vi "MyGraph-Facade.vi"(0 "Data In":T4, 2 "Display State In":T2, 3 "Container State":T3) -> (6 "Data Out":T4, 7 "Display State Out":T2, 8 "Action":T1)   [LabVIEW 2015, in "MyGraph.xctl"]
uses:
  MyGraph.xctl
  MyGraph-Data.ctl
  <vilib>/_xctls/Container State.ctl
  MyGraph-State.ctl
  <vilib>/_xctls/Action.ctl
  <vilib>/_xctls/XControlSupport.lvlib
panel:
  in  "ZoomREC":bool
  in  "ZoomToFit":bool
  in  "ZoomOut":bool
  in  "ZoomIn":bool
  in  "ZoomY":bool
  in  "ZoomX":bool
  in  "Select":bool
  out "Waveform Graph":waveform(dbl)[](graph)
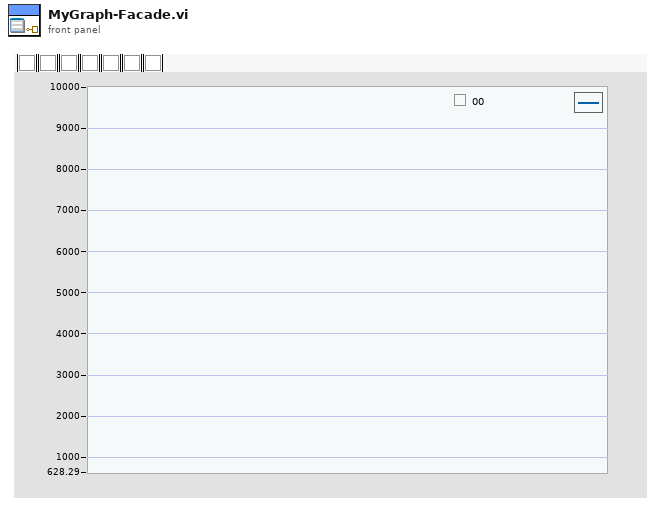
[diagram p1: front panel]
types:
  T1 = typedef "XControlSupport.lvlib/Action.ctl" = cluster{"Data Changed?":bool, "State Changed?":bool, "Action Name":string}
  T2 = typedef "MyGraph.xctl/MyGraph-State.ctl" = cluster{"PlotNames":string[], "event registration refnum":refnum<event-registration>}
  T3 = typedef "XControlSupport.lvlib/Container State.ctl" = cluster{"Indicator?":bool, "Run Mode?":bool, " Refnum":refnum<vi>}
  T4 = typedef "MyGraph.xctl/MyGraph-Data.ctl" = waveform(dbl)[]
  T5 = cluster{"ActTool":i32, "EmptyImg":picture, "StartPoints":cluster{i16, i16}[]}
  T6 = typedef "LVPoint32TypeDef.ctl" = cluster{"Horizontal":i32, "Vertical":i32}
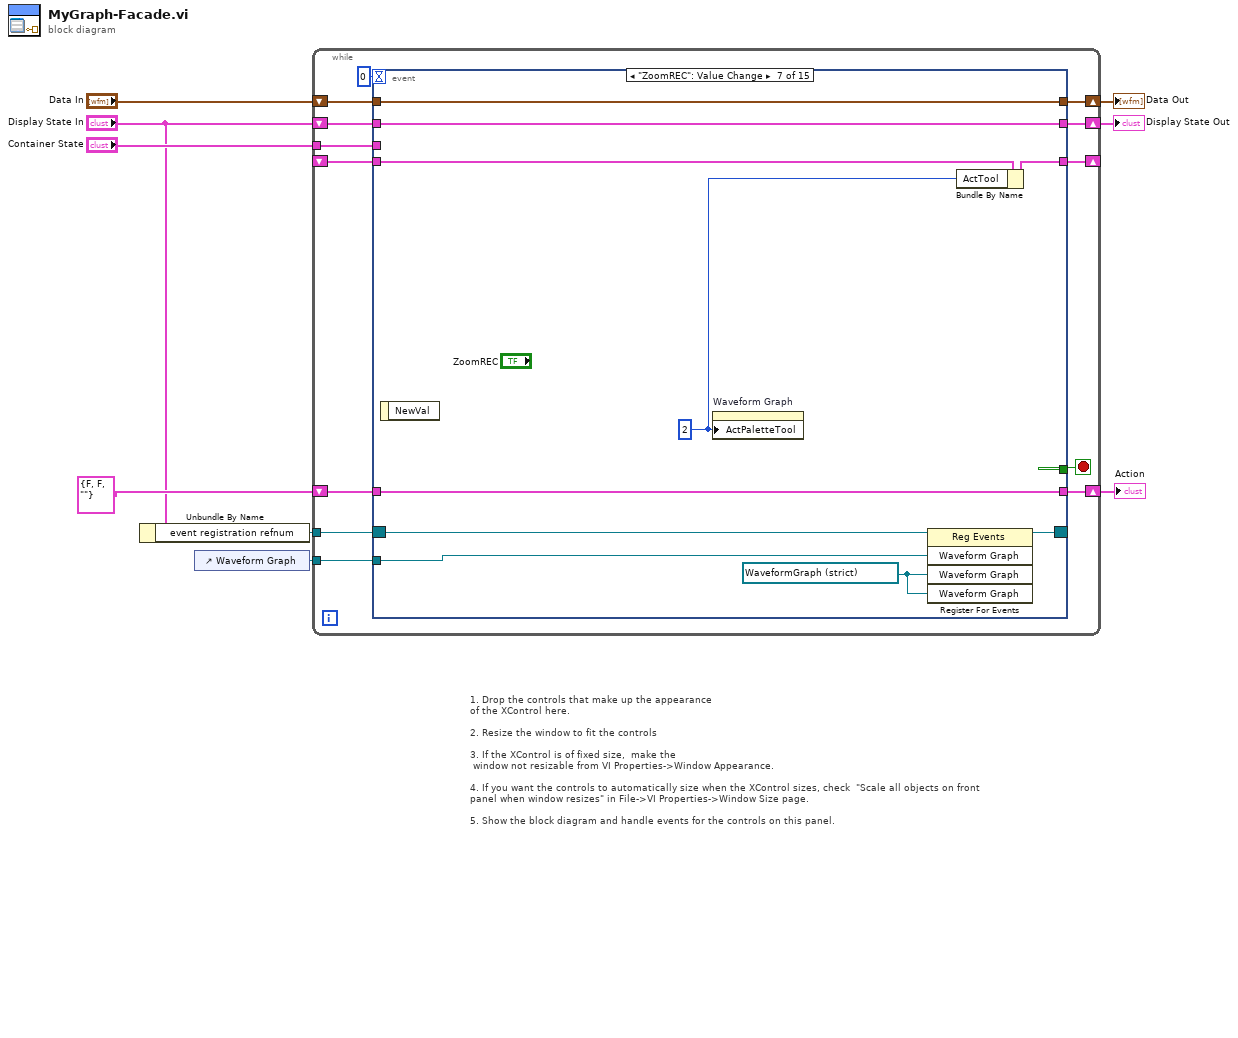
[diagram p0: block diagram]
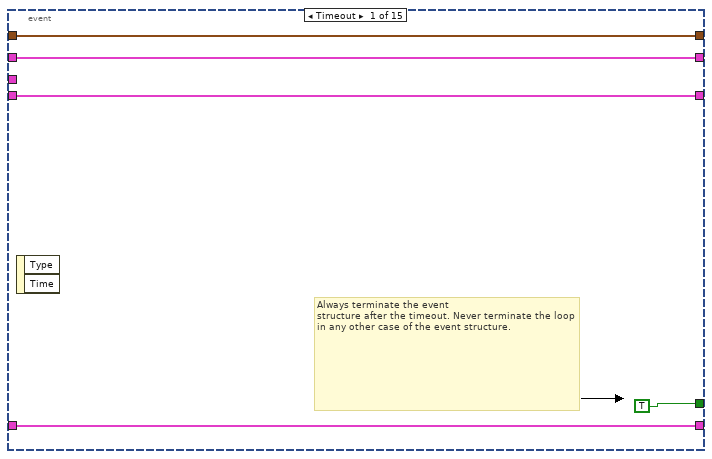
[diagram p2: hidden frame]
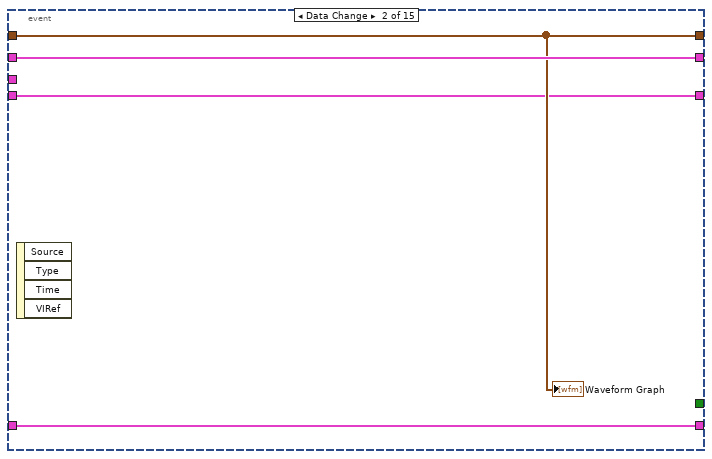
[diagram p3: hidden frame]
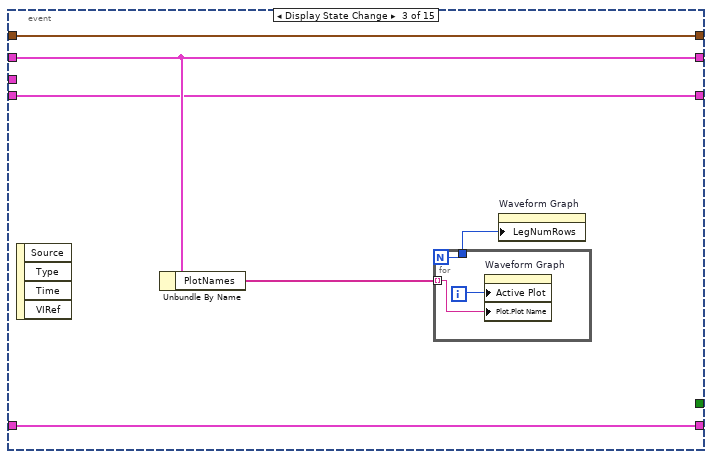
[diagram p4: hidden frame]
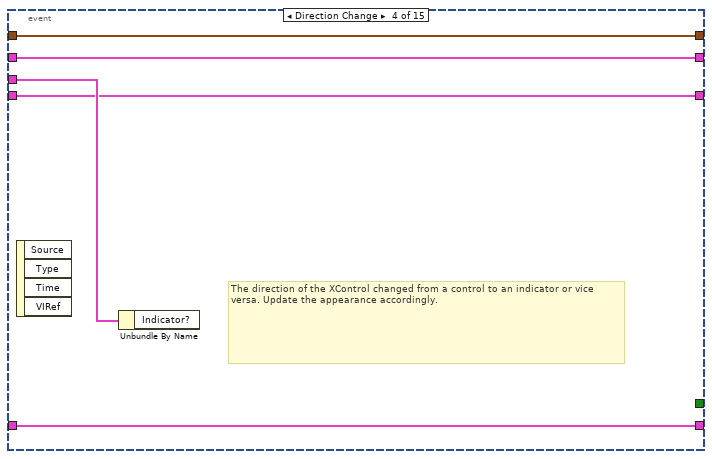
[diagram p5: hidden frame]
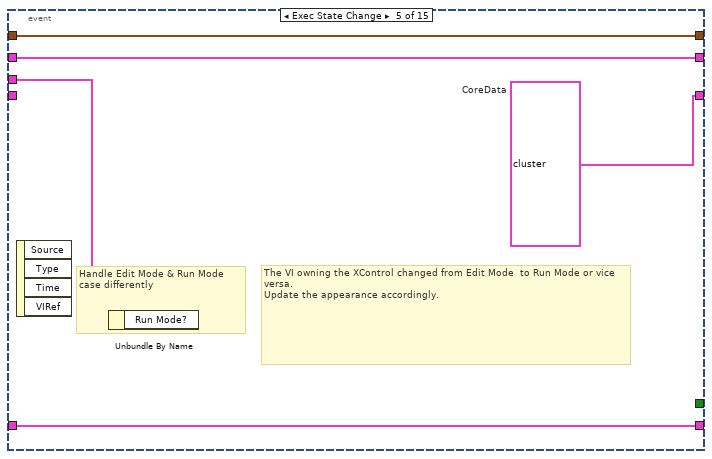
[diagram p6: hidden frame]
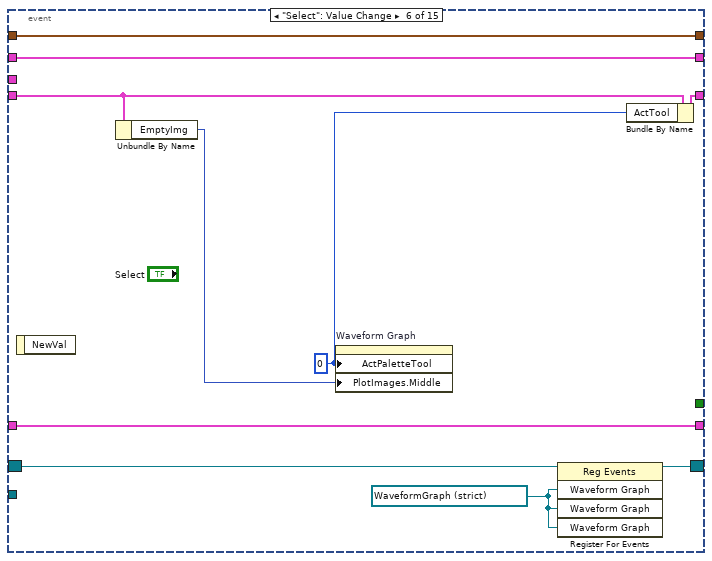
[diagram p7: hidden frame]
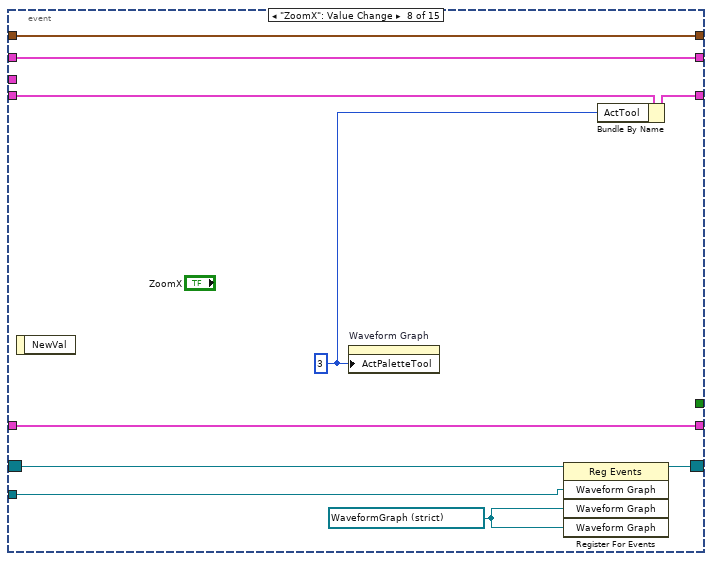
[diagram p8: hidden frame]
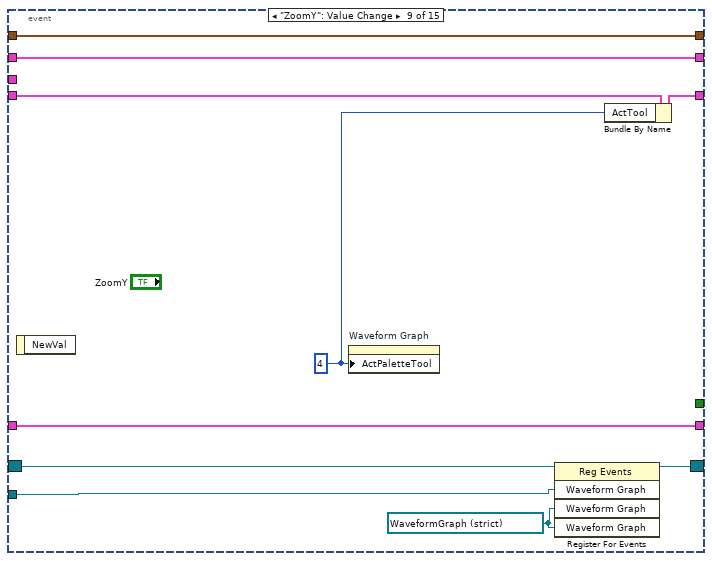
[diagram p9: hidden frame]
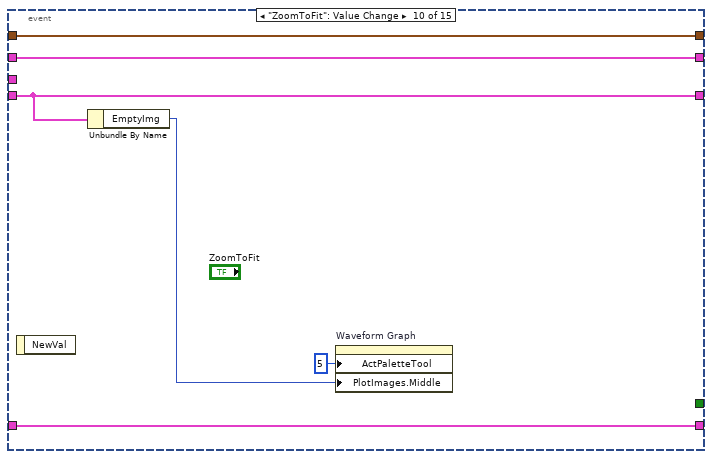
[diagram p10: hidden frame]
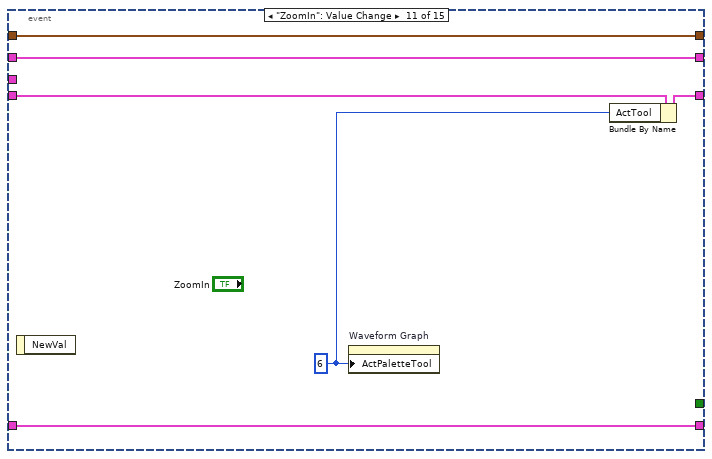
[diagram p11: hidden frame]
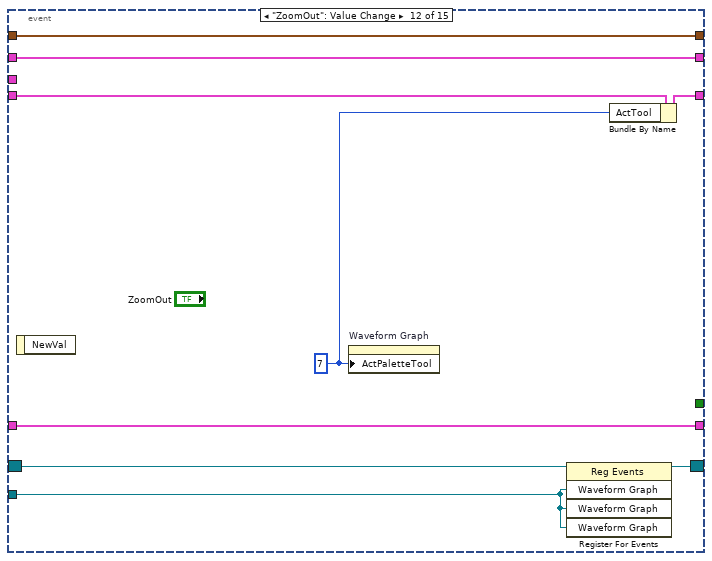
[diagram p12: hidden frame]
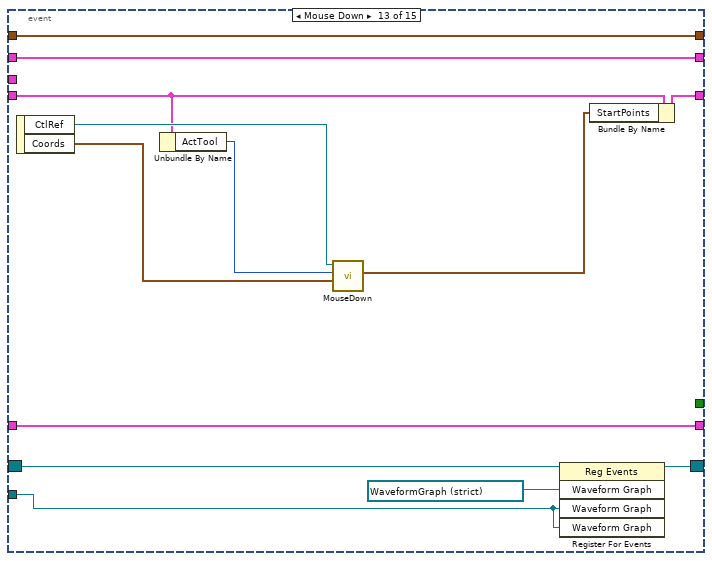
[diagram p13: hidden frame]
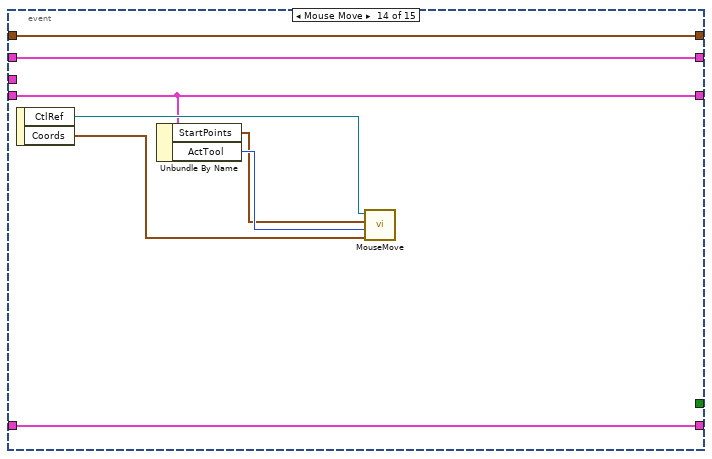
[diagram p14: hidden frame]
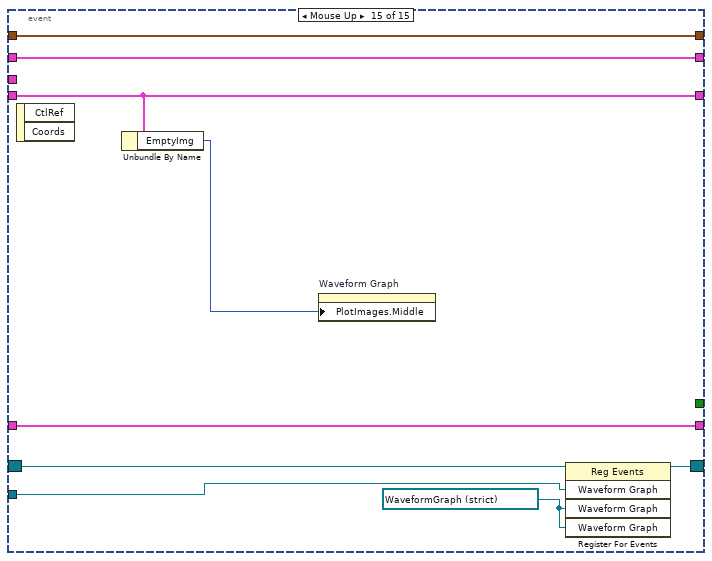
[diagram p15: hidden frame]
diagram:
  # "1. Drop the controls that make up the appearance\nof the XControl here.\n\n2. Resize the window to fit the controls\n\n3. If the XControl is of fixed size,  make the \n window not resizable from VI Properties->Window Appearance.\n\n4. If you want the controls to automatically size when the XControl sizes, check  \"Scale all objects on front panel when window resizes\" in File->VI Properties->Window Size page.\n\n5. Show the block diagram and handle events for the controls on this panel."
  n1 = Unbundle By Name("Display State In") -> ("event registration refnum"=w2:refnum<event-registration>)
  n2 = control-ref of="Waveform Graph"() -> (w1:refnum<vi>)
  n3 = while {
    shift-right: [w21] -> w6
    shift-left: "Display State In" -> [w22]
    tunnel: "Container State" -> [w18]
    shift-right: [w16] -> w9
    shift-left: "Data In" -> [w17]
    shift-right: [w14] -> w5
    shift-left: T1 {"Data Changed?"=FALSE, "State Changed?"=FALSE, "Action Name"=""} ("Action") -> [w15]
    tunnel: w2 -> [w13]
    shift-right: [w11] -> _
    shift-left: _ -> [w12]
    tunnel: w1 -> [w10]
    stop <- w20 stop-if-true
    n4 = event shown="[6] \"ZoomREC\": Value Change" {
      selector: w13 -> [_ _ _ _ _ w56 w65 w75 w85 _ _ w106 w114 _ w137]
      dyn-events: [_ _ _ _ _ w57 w66 w76 w86 _ _ w107 w115 _ w138] -> _
      timeout: 0 -> [_ _ _ _ _ _ _ _ _ _ _ _ _ _ _]
      tunnel: w22 -> [w25 w31 w35 w44 w49 w60 w70 w80 w90 w96 w102 w111 w124 w132 w141]
      tunnel: [w25 w31 w35 w44 w49 w60 w70 w80 w90 w96 w102 w111 w124 w132 w141] -> w21
      tunnel: [TRUE _ _ _ _ _ _ _ _ _ _ _ _ _ _] -> w20
      tunnel: w18 -> [_ _ _ w45 w50 _ _ _ _ _ _ _ _ _ _]
      tunnel: w17 -> [w24 w29 w37 w43 w48 w59 w69 w79 w89 w95 w101 w110 w123 w131 w140]
      tunnel: [w24 w29 w37 w43 w48 w59 w69 w79 w89 w95 w101 w110 w123 w131 w140] -> w16
      tunnel: [w26 w30 w36 w42 w47 w58 w68 w78 w88 w94 w100 w109 w122 w130 w139] -> w14
      tunnel: w15 -> [w26 w30 w36 w42 w47 w58 w68 w78 w88 w94 w100 w109 w122 w130 w139]
      tunnel: w12 -> [w23 w28 w32 w41 _ w52 w67 w77 w87 w92 w99 w108 w119 w127 w135]
      tunnel: [w23 w28 w32 w41 w46 w54 w63 w73 w83 w92 w98 w104 w117 w127 w135] -> w11
      tunnel: w10 -> [_ _ _ _ _ _ w64 w74 w84 _ _ w105 w112 _ w133]
      event Timeout {
        # "Always terminate the event\nstructure after the timeout. Never terminate the loop in any other case of the event structure."
        n5 = event-data() -> ()  [unwired: 1 in, 2 out]
      }
      event Data Change {
        n6 = event-data() -> ()  [unwired: 1 in, 4 out]
        "Waveform Graph" <- w29
      }
      event Display State Change {
        n7 = event-data() -> ()  [unwired: 1 in, 4 out]
        n8 = Unbundle By Name(w35) -> ("PlotNames"=w34:string[])
        n9 = for {
          N -> [w38]
          tunnel: w34 -> [w39] mode=indexing
          tunnel: [w38] -> w33
          i -> [w40]
          n10 = property on="Waveform Graph" class="WFGraph (strict)"("Active Plot"=w40, "Plot.Plot Name"=w39) -> ()  [unwired: 2 in, 2 out]
        }
        n11 = property on="Waveform Graph" class="WFGraph (strict)"("LegNumRows"=w33) -> ()  [unwired: 2 in, 2 out]
      }
      event Direction Change {
        # "The direction of the XControl changed from a control to an indicator or vice versa. Update the appearance accordingly."
        n12 = event-data() -> ()  [unwired: 1 in, 4 out]
        n13 = Unbundle By Name(w45) -> ()  [unwired: 1 out]
      }
      event Exec State Change {
        w46 = T5 {"ActTool"=0, "EmptyImg"=bytes[0], "StartPoints"=[]}  # CoreData
        # "The VI owning the XControl changed from Edit Mode  to Run Mode or vice versa.\nUpdate the appearance accordingly."
        # "Handle Edit Mode & Run Mode\ncase differently"
        n14 = event-data() -> ()  [unwired: 1 in, 4 out]
        n15 = Unbundle By Name(w50) -> ()  [unwired: 1 out]
      }
      event "Select": Value Change {
        w55 = refnum<vi> refnum ("Waveform Graph")
        w53 = 0 ("Palette:Active Tool")
        n16 = event-data() -> ()  [unwired: 1 in, 1 out]
        n17 = Unbundle By Name(w52) -> ("EmptyImg"=w51:picture)
        n18 = property on="Waveform Graph" class="WFGraph (strict)"("ActPaletteTool"=w53, "PlotImages.Middle"=w51) -> ()  [unwired: 2 in, 2 out]
        n19 = register-events(reference=w56, w55, w55, w55) -> (reference out=w57:refnum<event-registration>)  [unwired: 1 in, 1 out]
        n20 = Bundle By Name(cluster=w52, "ActTool"=w53) -> (w54:T5)
      }
      event "ZoomREC": Value Change {
        w61 = refnum<vi> refnum ("Waveform Graph")
        w62 = 2 ("Palette:Active Tool")
        n21 = event-data() -> ()  [unwired: 1 in, 1 out]
        n22 = property on="Waveform Graph" class="WFGraph (strict)"("ActPaletteTool"=w62) -> ()  [unwired: 2 in, 2 out]
        n23 = register-events(reference=w65, w64, w61, w61) -> (reference out=w66:refnum<event-registration>)  [unwired: 1 in, 1 out]
        n24 = Bundle By Name(cluster=w67, "ActTool"=w62) -> (w63:T5)
      }
      event "ZoomX": Value Change {
        w71 = refnum<vi> refnum ("Waveform Graph")
        w72 = 3 ("Palette:Active Tool")
        n25 = event-data() -> ()  [unwired: 1 in, 1 out]
        n26 = property on="Waveform Graph" class="WFGraph (strict)"("ActPaletteTool"=w72) -> ()  [unwired: 2 in, 2 out]
        n27 = register-events(reference=w75, w74, w71, w71) -> (reference out=w76:refnum<event-registration>)  [unwired: 1 in, 1 out]
        n28 = Bundle By Name(cluster=w77, "ActTool"=w72) -> (w73:T5)
      }
      event "ZoomY": Value Change {
        w81 = refnum<vi> refnum ("Waveform Graph")
        w82 = 4 ("Palette:Active Tool")
        n29 = event-data() -> ()  [unwired: 1 in, 1 out]
        n30 = property on="Waveform Graph" class="WFGraph (strict)"("ActPaletteTool"=w82) -> ()  [unwired: 2 in, 2 out]
        n31 = register-events(reference=w85, w84, w81, w81) -> (reference out=w86:refnum<event-registration>)  [unwired: 1 in, 1 out]
        n32 = Bundle By Name(cluster=w87, "ActTool"=w82) -> (w83:T5)
      }
      event "ZoomToFit": Value Change {
        n33 = event-data() -> ()  [unwired: 1 in, 1 out]
        n34 = Unbundle By Name(w92) -> ("EmptyImg"=w91:picture)
        n35 = property on="Waveform Graph" class="WFGraph (strict)"("ActPaletteTool"=5 ("Palette:Active Tool"), "PlotImages.Middle"=w91) -> ()  [unwired: 2 in, 2 out]
      }
      event "ZoomIn": Value Change {
        w97 = 6 ("Palette:Active Tool")
        n36 = event-data() -> ()  [unwired: 1 in, 1 out]
        n37 = property on="Waveform Graph" class="WFGraph (strict)"("ActPaletteTool"=w97) -> ()  [unwired: 2 in, 2 out]
        n38 = Bundle By Name(cluster=w99, "ActTool"=w97) -> (w98:T5)
      }
      event "ZoomOut": Value Change {
        w103 = 7 ("Palette:Active Tool")
        n39 = event-data() -> ()  [unwired: 1 in, 1 out]
        n40 = property on="Waveform Graph" class="WFGraph (strict)"("ActPaletteTool"=w103) -> ()  [unwired: 2 in, 2 out]
        n41 = register-events(reference=w106, w105, w105, w105) -> (reference out=w107:refnum<event-registration>)  [unwired: 1 in, 1 out]
        n42 = Bundle By Name(cluster=w108, "ActTool"=w103) -> (w104:T5)
      }
      event Mouse Down {
        n43 = event-data() -> ("CtlRef"=w121:refnum<vi>, "Coords"=w120:T6)  [unwired: 1 in]
        n44 = Unbundle By Name(w119) -> ("ActTool"=w118:i32)
        n45 = call "MouseDown.vi"("Coords"=w120, "ActTool"=w118, "reference"=w121) -> ("StartPoints"=w116:cluster{i16, i16}[])  [unwired: 7 in, 1 out]
        n46 = register-events(reference=w114, refnum<vi> refnum ("Waveform Graph"), w112, w112) -> (reference out=w115:refnum<event-registration>)  [unwired: 1 in, 1 out]
        n47 = Bundle By Name(cluster=w119, "StartPoints"=w116) -> (w117:T5)
      }
      event Mouse Move {
        n48 = event-data() -> ("CtlRef"=w129:refnum<vi>, "Coords"=w128:T6)  [unwired: 1 in]
        n49 = Unbundle By Name(w127) -> ("StartPoints"=w125:cluster{i16, i16}[], "ActTool"=w126:i32)
        n50 = call "MouseMove.vi"("Coords"=w128, "ActTool"=w126, "StartPoints"=w125, "reference"=w129) -> ()  [unwired: 8 in]
      }
      event Mouse Up {
        w136 = refnum<vi> refnum ("Waveform Graph")
        n51 = event-data() -> ()  [unwired: 1 in, 2 out]
        n52 = Unbundle By Name(w135) -> ("EmptyImg"=w134:picture)
        n53 = property on="Waveform Graph" class="WFGraph (strict)"("PlotImages.Middle"=w134) -> ()  [unwired: 2 in, 2 out]
        n54 = register-events(reference=w137, w133, w136, w136) -> (reference out=w138:refnum<event-registration>)  [unwired: 1 in, 1 out]
      }
    }
  }
  "Display State Out" <- w6
  "Data Out" <- w9
  "Action" <- w5
